vi "UHR-Fleezers Control (host) - 12.1_Jonathan.vi"() -> ()   [LabVIEW 2012] (continued)
          tunnel: [w1121] -> w1086
          tunnel: w1085 -> [w1121]
          tunnel: [w1125] -> w1087
          tunnel: w1086 -> [w1125]
          tunnel: w1087 -> [w1127]
          frame #0 {
            n678 = property on="Trap Delta (MHz)" class="DigNum (strict)"("Val(Sgnl)"="Trap Delta Before Moving") -> ()  [unwired: 2 in, 2 out]
          }
          frame #1 {
            n679 = local read "Saved Stage Positions"() -> (w1098:dbl[][])
            n680 = local write "FB Trap Pos Offset"(0.0 ("FB Trap Pos Offset")) -> ()
            n681 = property on="Trap Pos. FB Offset Factor" class="DigNum (strict)"("Val(Sgnl)"=i64 0 ("Value (Signaling)")) -> ()  [unwired: 2 in, 2 out]
            n682 = local write "Stage Moving"(TRUE ("Stage Moving")) -> ()
            n683 = call "move to saved stage position.vi"("error in"=w1095, "Stage VISA resource name in"=w1096, "Position"="Stage Position To Establish FB", "Saved Stage Positions"=w1098) -> ("error out"=w1094:errorcluster)  [unwired: 1 out]
            n684 = local write "Stage Control Serial Error"(w1094) -> ()
          }
          frame #2 {
            n685 = call <vilib>:"Beep.vi"() -> ()  [unwired: 3 in, 9 out]
            n686 = Multiply(x="Wait (s)", y=u32 1000 ("milliseconds to wait")) -> (x*y=w1104:u32)
            n687 = property on="Trap Delta (MHz)" class="DigNum (strict)"("Val(Sgnl)"="Starting \nTrap Delta (MHz)") -> ()  [unwired: 2 in, 2 out]
            n688 = local write "Stage Moving"(FALSE ("Stage Moving")) -> ()
            n689 = Wait (ms)(milliseconds to wait=w1104) -> ()  [unwired: 1 out]
            n690 = property on="Tab Control 2" class="TabCtl (strict)"("Val(Sgnl)"=T7."Feedback on Trap Position" ("Value (Signaling)")) -> ()  [unwired: 2 in, 2 out]
            n691 = property on="Tab Control" class="TabCtl (strict)"("Val(Sgnl)"=T27."Trap Control (RF)" ("Value (Signaling)")) -> ()  [unwired: 2 in, 2 out]
          }
          frame #3 {
            n692 = property on="Set Reading to\nSetpoint" class="Bool (strict)"("Val(Sgnl)"=TRUE ("Value (Signaling)")) -> ()  [unwired: 2 in, 2 out]
            n693 = Wait (ms)(milliseconds to wait=u32 500) -> ()  [unwired: 1 out]
          }
          frame #4 {
            n694 = property on="Trap Pos. FB ON" class="Bool (strict)"("Val(Sgnl)"=TRUE ("Value (Signaling)")) -> ()  [unwired: 2 in, 2 out]
            n695 = Wait (ms)(milliseconds to wait=u32 250) -> ()  [unwired: 1 out]
          }
          frame #5 {
            n696 = case shown="False" "Trap Trig Fl." {
              frame False {
                n697 = case shown="True" "Green ON after FB ON?" {
                  selector: "Green ON after FB ON?" -> [_ w1120]
                  frame False {
                  }
                  frame True {
                    n698 = property on="Green Laser ON/Interlacing" class="Bool (strict)"("Val(Sgnl)"=w1120) -> ()  [unwired: 2 in, 2 out]
                  }
                }
              }
              frame True {
              }
            }
            n699 = case shown="True" "Remove Action Offset" {
              tunnel: TRUE ("Value (Signaling)") -> [w1117 w1118]
              frame False {
                n700 = property on="Remove Unwinding Offset" class="Bool (strict)"("Val(Sgnl)"=w1117) -> ()  [unwired: 2 in, 2 out]
              }
              frame True {
                n701 = property on="Remove Action Offset" class="Bool (strict)"("Val(Sgnl)"=w1118) -> ()  [unwired: 2 in, 2 out]
              }
            }
            n702 = Wait (ms)(milliseconds to wait=u32 250) -> ()  [unwired: 1 out]
          }
          frame #6 {
            n703 = property on="Start Saving" class="Bool (strict)"("Val(Sgnl)"=TRUE ("Value (Signaling)")) -> ()  [unwired: 2 in, 2 out]
            n704 = Wait (ms)(milliseconds to wait=u32 5000) -> ()  [unwired: 1 out]
          }
          frame #7 {
            w1124 = TRUE ("Value (Signaling)")
            n705 = property on="Rem fb disp offset" class="Bool (strict)"("Val(Sgnl)"=w1124) -> ()  [unwired: 2 in, 2 out]
            n706 = property on="Remove Offset" class="Bool (strict)"("Val(Sgnl)"=w1124) -> ()  [unwired: 2 in, 2 out]
            n707 = Wait (ms)(milliseconds to wait=u32 100) -> ()  [unwired: 1 out]
          }
          frame #8 {
            n708 = case shown="True" w1127 {
              frame False {
              }
              frame True {
                n709 = local write "Trap Trig. Fl."(TRUE ("Value (Signaling)")) -> ()
              }
            }
          }
          frame #9 {
            n710 = case shown="True" "Start dipping after?" {
              frame False {
              }
              frame True {
                n711 = flat-sequence {
                  frame #0 {
                    n712 = Multiply(x="Delay before dipping (s)", y=1000.0) -> (x*y=w1131:dbl)
                    n713 = Wait (ms)(milliseconds to wait=w1131) -> ()  [unwired: 1 out]
                  }
                  frame #1 {
                    n714 = property on="Dip for Protein" class="Bool (strict)"("Val(Sgnl)"=TRUE ("Value (Signaling)")) -> ()  [unwired: 2 in, 2 out]
                    n715 = local write "Scripts"(T2."Dipping" ("Scripts")) -> ()
                  }
                }
              }
            }
          }
        }
      }
      event "Fixed Traps Data\nScript": Value Change {
        n716 = event-data() -> ()  [unwired: 1 in, 5 out]
        n717 = flat-sequence {
          frame #0 {
            n718 = case shown="True" "Green ON" {
              frame False {
              }
              frame True {
                n719 = property on="Green Laser ON/Interlacing" class="Bool (strict)"("Val(Sgnl)"=TRUE) -> ()  [unwired: 2 in, 2 out]
              }
            }
            n720 = local write "Offset (nm)"(0.0 ("Offset (nm)")) -> ()
            n721 = property on="Sample Channel\nFlow" class="Bool (strict)"("Val(Sgnl)"=FALSE ("Value (Signaling)")) -> ()  [unwired: 2 in, 2 out]
            n722 = property on="Trap Delta (MHz)" class="DigNum (strict)"("Val(Sgnl)"="Fixed Traps Trap Delta (MHz)") -> ()  [unwired: 2 in, 2 out]
          }
          frame #1 {
            n723 = Wait (ms)(milliseconds to wait=u32 1000) -> ()  [unwired: 1 out]
          }
          frame #2 {
            n724 = local write "Start Saving"(TRUE ("Start Saving")) -> ()
          }
          frame #3 {
            n725 = local read "Bead Sep. Int. Time (s)"() -> (w1142:dbl)
            n726 = Multiply(x=w1142, y=1000.0) -> (x*y=w1144:dbl)
            n727 = Wait (ms)(milliseconds to wait=w1144) -> ()  [unwired: 1 out]
          }
          frame #4 {
            n728 = property on="Remove Offset" class="Bool (strict)"("Val(Sgnl)"=TRUE ("Value (Signaling)")) -> ()  [unwired: 2 in, 2 out]
          }
          frame #5 {
            n729 = property on="Dip for Protein" class="Bool (strict)"("Val(Sgnl)"="Start dipping after?") -> ()  [unwired: 2 in, 2 out]
          }
        }
      }
      event "Got DNA bead": Value Change {
        n730 = event-data() -> ()  [unwired: 1 in, 5 out]
        n731 = flat-sequence {
          frame #0 {
            n732 = local read "Daq spot flow on"() -> (w1149:bool)
            n733 = case shown="True" w1149 {
              frame False {
              }
              frame True {
                n734 = property on="Sample Channel\nFlow" class="Bool (strict)"("Val(Sgnl)"=TRUE ("Value (Signaling)")) -> ()  [unwired: 2 in, 2 out]
              }
            }
            n735 = property on="Got DNA bead" class="Bool"("Key Focus"=FALSE) -> ()  [unwired: 2 in, 2 out]
          }
          frame #1 {
            n736 = property on="Inject Pump 1" class="Bool (strict)"("Val(Sgnl)"=FALSE ("Value (Signaling)")) -> ()  [unwired: 2 in, 2 out]
          }
          frame #2 {
            n737 = property on="Cal/Data Acq. Spot" class="Bool (strict)"("Val(Sgnl)"=TRUE ("Value (Signaling)")) -> ()  [unwired: 2 in, 2 out]
          }
        }
      }
      event "Take Stepping Data": Value Change {
        n738 = event-data() -> ()  [unwired: 1 in, 5 out]
        n739 = local read "Save ave N"() -> (w1161:dbl)
        n740 = flat-sequence {
          tunnel: w1161 -> [w1163]
          tunnel: [w1163] -> w1156
          tunnel: [w1165] -> w1157
          tunnel: w1156 -> [w1165]
          tunnel: [w1167] -> w1158
          tunnel: w1157 -> [w1167]
          tunnel: [w1170] -> w1159
          tunnel: w1158 -> [w1170]
          tunnel: [w1172] -> w1160
          tunnel: w1159 -> [w1172]
          tunnel: [w1174] -> w1154
          tunnel: w1160 -> [w1174]
          tunnel: w1154 -> [w1177]
          tunnel: [w1177] -> w1153
          tunnel: w1153 -> [w1178]
          tunnel: [w1178] -> w1155
          tunnel: w1155 -> [w1184]
          frame #0 {
            n741 = property on="Save ave N" class="DigNum (strict)"("Val(Sgnl)"="Save ave factor") -> ()  [unwired: 2 in, 2 out]
          }
          frame #1 {
            n742 = Wait (ms)(milliseconds to wait=u32 100) -> ()  [unwired: 1 out]
          }
          frame #2 {
            n743 = local read "Offset 2 Start (MHz)"() -> (w1169:dbl)
            n744 = property on="Saved AOD Raster Scan Parameter Sets" class="Arr (strict)"("Index Values"=u32[] [2]) -> ()  [unwired: 2 in, 2 out]
            n745 = property on="Trap Delta (MHz)" class="DigNum (strict)"("Val(Sgnl)"=w1169) -> ()  [unwired: 2 in, 2 out]
          }
          frame #3 {
            n746 = property on="Load parameters" class="Bool (strict)"("Val(Sgnl)"=TRUE ("Value (Signaling)")) -> ()  [unwired: 2 in, 2 out]
          }
          frame #4 {
            n747 = Wait (ms)(milliseconds to wait=u32 100) -> ()  [unwired: 1 out]
          }
          frame #5 {
            n748 = property on="Trap Raster Scan" class="Bool (strict)"("Val(Sgnl)"=TRUE ("Value (Signaling)")) -> ()  [unwired: 2 in, 2 out]
          }
          frame #6 {
            n749 = Wait (ms)(milliseconds to wait=u32 1000) -> ()  [unwired: 1 out]
          }
          frame #7 {
            n750 = while {
              stop <- w1181 stop-if-true
              n751 = local read "Raster Scanning..."() -> (w1183:bool)
              n752 = local read "Saving..."() -> (w1182:bool)
              n753 = Not(x=w1182) -> (.not. x?=w1179:bool)
              n754 = Not(x=w1183) -> (.not. x?=w1180:bool)
              n755 = And(x=w1180, y=w1179) -> (x .and. y?=w1181:bool)
            }
          }
          frame #8 {
            n756 = property on="Save ave N" class="DigNum (strict)"("Val(Sgnl)"=w1184) -> ()  [unwired: 2 in, 2 out]
          }
        }
      }
      event "Step Size (nm)": Value Change {
        n757 = event-data() -> ()  [unwired: 1 in, 5 out]
        n758 = flat-sequence {
          frame #0 {
            n759 = property on="Saved AOD Raster Scan Parameter Sets" class="Arr (strict)"("Index Values"=u32[] [1]) -> ()  [unwired: 2 in, 2 out]
          }
          frame #1 {
            n760 = Multiply(x="N Steps", y="Step Size (nm)") -> (x*y=w1186:dbl)
            n761 = property on="Scan Speed AOD (nm/s) 2" class="DigNum (strict)"("Value"="Step Size (nm)") -> ()  [unwired: 2 in, 2 out]
            n762 = property on="Step Size AOD (nm) 2" class="DigNum (strict)"("Value"="Step Size (nm)") -> ()  [unwired: 2 in, 2 out]
            n763 = property on="Scan Range AOD (nm) 2" class="DigNum (strict)"("Value"=w1186) -> ()  [unwired: 2 in, 2 out]
          }
        }
      }
      event "Take Detection Laser\nImage": Value Change {
        n764 = event-data() -> ()  [unwired: 1 in, 5 out]
        n765 = flat-sequence {
          tunnel: [w1214] -> w1204
          tunnel: [w1213] -> w1197
          tunnel: [w1212] -> w1189
          tunnel: [w1217] -> w1205
          tunnel: w1204 -> [w1217]
          tunnel: [w1216] -> w1198
          tunnel: w1197 -> [w1216]
          tunnel: [w1215] -> w1190
          tunnel: w1189 -> [w1215]
          tunnel: [w1221] -> w1206
          tunnel: w1205 -> [w1221]
          tunnel: [w1220] -> w1199
          tunnel: w1198 -> [w1220]
          tunnel: [w1219] -> w1191
          tunnel: w1190 -> [w1219]
          tunnel: [w1227] -> w1207
          tunnel: w1206 -> [w1227]
          tunnel: [w1226] -> w1200
          tunnel: w1199 -> [w1226]
          tunnel: [w1225] -> w1192
          tunnel: w1191 -> [w1225]
          tunnel: [w1231] -> w1208
          tunnel: w1207 -> [w1231]
          tunnel: [w1230] -> w1201
          tunnel: w1200 -> [w1230]
          tunnel: [w1229] -> w1193
          tunnel: w1192 -> [w1229]
          tunnel: [w1235] -> w1209
          tunnel: w1208 -> [w1235]
          tunnel: [w1234] -> w1202
          tunnel: w1201 -> [w1234]
          tunnel: [w1233] -> w1194
          tunnel: w1193 -> [w1233]
          tunnel: [w1239] -> w1210
          tunnel: w1209 -> [w1239]
          tunnel: [w1238] -> w1203
          tunnel: w1202 -> [w1238]
          tunnel: [w1237] -> w1195
          tunnel: w1194 -> [w1237]
          tunnel: w1210 -> [w1245]
          tunnel: w1203 -> [w1244]
          tunnel: [w1242] -> w1196
          tunnel: w1195 -> [w1242]
          tunnel: w1196 -> [w1246]
          frame #0 {
            n766 = local read "Green Laser ON/Interlacing"() -> (w1214:bool)
            n767 = local read "Green laser mode"() -> (w1213:enum32{"Laser ON", "Laser OFF", "Interlace"})
            n768 = local read "Green FB On/Off"() -> (w1212:bool)
          }
          frame #1 {
            n769 = property on="Green FB On/Off" class="Bool (strict)"("Val(Sgnl)"=FALSE ("Value (Signaling)")) -> ()  [unwired: 2 in, 2 out]
          }
          frame #2 {
            n770 = property on="Green Laser ON/Interlacing" class="Bool (strict)"("Val(Sgnl)"=TRUE ("Value (Signaling)")) -> ()  [unwired: 2 in, 2 out]
            n771 = property on="Flip Green Filter" class="Bool (strict)"("Val(Sgnl)"=TRUE ("Value (Signaling)")) -> ()  [unwired: 2 in, 2 out]
            n772 = property on="Green laser mode" class="RadioBtnsControl (strict)"("Val(Sgnl)"=enum32{"Laser ON", "Laser OFF", "Interlace"}."Laser ON" ("Value (Signaling)")) -> ()  [unwired: 2 in, 2 out]
          }
          frame #3 {
            n773 = Wait (ms)(milliseconds to wait=u32 500) -> ()  [unwired: 1 out]
          }
          frame #4 {
            n774 = property on="Confocal Image" class="Bool (strict)"("Val(Sgnl)"=TRUE ("Value (Signaling)")) -> ()  [unwired: 2 in, 2 out]
          }
          frame #5 {
            n775 = Wait (ms)(milliseconds to wait=u32 2000) -> ()  [unwired: 1 out]
          }
          frame #6 {
            n776 = while {
              stop <- w1240 stop-if-true
              n777 = local read "Saving..."() -> (w1241:bool)
              n778 = Not(x=w1241) -> (.not. x?=w1240:bool)
            }
          }
          frame #7 {
            n779 = property on="Flip Green Filter" class="Bool (strict)"("Val(Sgnl)"=TRUE ("Value (Signaling)")) -> ()  [unwired: 2 in, 2 out]
            n780 = property on="Green Laser ON/Interlacing" class="Bool (strict)"("Val(Sgnl)"=w1245) -> ()  [unwired: 2 in, 2 out]
            n781 = property on="Green laser mode" class="RadioBtnsControl (strict)"("Val(Sgnl)"=w1244) -> ()  [unwired: 2 in, 2 out]
          }
          frame #8 {
            n782 = property on="Green FB On/Off" class="Bool (strict)"("Val(Sgnl)"=w1246) -> ()  [unwired: 2 in, 2 out]
          }
        }
      }
      event "Stop All": Value Change {
        n783 = event-data() -> ()  [unwired: 1 in, 5 out]
        n784 = local read "Stop All"() -> (w1247:bool)
      }
    }
    n785 = node-c288() -> ()  [unwired: 1 in, 1 out]
  }
  n786 = node-c288(3 ("Processor")) -> (w97:T22)  [unwired: 3 out]
  n787 = flat-sequence "Video" {
    tunnel: [w1257] -> w87
    tunnel: w87 -> [w1297]
    frame #0 {
      n788 = while {
        stop <- w1249 continue-if-true
        n789 = call "Close Video Capture.vi"() -> ("error code OUT"=w1251:i32)
        n790 = Equal?(x=w1251, y=0) -> (x = y?=w1249:bool)
      }
      n791 = local write "Stop All"(FALSE ("Stop All")) -> ()
    }
    frame #1 {
      n792 = call "DMR_Init.vi"() -> ()  [unwired: 3 out]
    }
    frame #2 {
      w1252 = "DE245428202"  # MSU fleezers card #
      (unwired) "DE019116701"  # Illinois fleezers card #
      # "Setting the destination format to Mono8 makes sure that the image can be displayed in the intensity plot."
      n793 = call "DMR_GetDevice.vi"("search string IN"=w1252) -> ("device handle OUT"=w1275:i32)  [unwired: 4 in, 2 out]
      n794 = call "DMR_OpenDevice.vi"("device handle IN"=w1275) -> ("driver handle OUT"=w1258:i32)  [unwired: 4 out]
      n795 = call "DMR_FindList.vi"("flags IN"=u32 0 ("flags"), "list name IN"="" ("String"), "list type IN"=T28."camera descriptions", "driver handle IN"=w1258) -> ("list handle OUT"=w1261:i32)  [unwired: 2 out]
      n796 = call "DMR_FindList.vi"("flags IN"=u32 0 ("flags"), "list name IN"="Base", "list type IN"=T28."setting", "driver handle IN"=w1258) -> ("list handle OUT"=w1259:i32)  [unwired: 2 out]
      n797 = call "OBJ_GetHandle.vi"("object name IN"="VideoStandard", "list handle IN"=w1261) -> ("object handle OUT"=w1255:i32)  [unwired: 3 out]
      n798 = call "OBJ_GetHandle.vi"("object name IN"="PixelFormat", "list handle IN"=w1259) -> ("object handle OUT"=w1269:i32)  [unwired: 3 out]
      n799 = call "OBJ_SetS.vi"("value index IN"=0, "value IN"="NTSC M", "object handle IN"=w1255) -> ()  [unwired: 2 out]
      n800 = call "OBJ_SetS.vi"("value index IN"=0, "value IN"="Mono8" ("value"), "object handle IN"=w1269) -> ()  [unwired: 2 out]
      n801 = call "OBJ_GetHandle.vi"("object name IN"="VideoChannel", "list handle IN"=w1259) -> ("object handle OUT"=w1265:i32)  [unwired: 3 out]
      n802 = while {
        tunnel: [w1279] -> w1257
        tunnel: w1258 -> [w1276]
        stop <- w1277 continue-if-true
        n803 = call "DMR_ImageRequestSingle.vi"("request control IN"=0, "driver handle IN"=w1276) -> ("error code OUT"=w1278:i32, "driver handle OUT"=w1279:i32)  [unwired: 2 out]
        n804 = Equal To 0?(x=w1278) -> (x = 0?=w1277:bool)
      }
      n805 = call "OBJ_SetI.vi"("value index IN"=0, "value IN"=3 ("Video channel"), "object handle IN"=w1265) -> ()  [unwired: 2 out]
    }
    frame #3 {
      w1285 = T18 0 items=["Grayscale (U8)", "Grayscale (I16)", "Grayscale (SGL)", "Complex (CSG)", "RGB (U32)", "HSL (U32)", "RGB (U64)"] ("Image Type")
      w1293 = T18 0 items=["Grayscale (U8)", "Grayscale (I16)", "Grayscale (SGL)", "Complex (CSG)", "RGB (U32)", "HSL (U32)", "RGB (U64)"] ("Image Type")
      n806 = for "Create Greyscale map" {
        N: 256 -> [_]
        tunnel: [w1299] -> w1282 mode=indexing
        workers-P: _ -> [_]
        i -> [w1302]
        n807 = To Unsigned Byte Integer(number=w1302) -> (unsigned 8bit integer=w1298:u8)
        n808 = Join Numbers(hi=w1298, lo=w1298) -> ((hi.lo)=w1301:u16)
        n809 = Join Numbers(hi=w1298, lo=w1298) -> ((hi.lo)=w1300:u16)
        n810 = Join Numbers(hi=w1301, lo=w1300) -> ((hi.lo)=w1299:u32)
      }
      n811 = call "IMAQ Create"("Image Name"="Scaled video", "Image Type"=w1285) -> ("New Image"=w1284:T3)  [unwired: 2 in, 2 out]
      n812 = call "IMAQ Create"("Image Name"="Main video", "Image Type"=w1293) -> ("New Image"=w1294:T3)  [unwired: 2 in, 2 out]
      n813 = node-c288(0 ("Processor")) -> (w1292:T22)  [unwired: 3 out]
      n814 = Initialize Array(u32 0 ("Window Number (0...15)"), 480 ("dimension size"), 640 ("dimension size")) -> (w1287:u32[][])
      n815 = timed-loop {
        tunnel: w1297 -> [w1319]
        tunnel: [w1318] -> w1296
        tunnel: w1294 -> [w1317]
        timing: w1292 -> [_]
        timing-out: [_] -> w1291
        tunnel: w1287 -> [w1306]
        tunnel: w1284 -> [w1304]
        tunnel: w1282 -> [w1303]
        stop <- w1305 stop-if-true
        # "This block performs the \nactual image capture."
        n816 = node-c288() -> ()  [unwired: 2 out]
        n817 = local read "Stop All"() -> (w1305:bool)
        n818 = Reciprocal(x="Video Capture Rate (Hz)") -> (1/x=w1309:dbl)
        n819 = Multiply(x=w1309, y=1000.0) -> (x*y=w1307:dbl)
        n820 = call "DMR_ImageRequestWaitFor.vi"("queue number IN"=0, "timeout(ms) IN"=500, "driver handle IN"=w1319) -> ("error code OUT"=w1323:i32, "request number OUT"=w1320:i32, "driver handle OUT"=w1321:i32)
        n821 = feedback #1(T29 refnum ("Avi Refnum")) -> (w1311:T29)
        n822 = case shown="True" "New Video File" {
          tunnel: [T29 refnum ("Avi Refnum") w1340] -> w1313
          tunnel: [FALSE TRUE] -> w1314
          tunnel: w1311 -> [_ w1336]
          frame False {
          }
          frame True {
            n823 = call "Create new save file.vi"("Ext"=".avi" ("string"), "Index In"="Video Index") -> ("Path Out"=w1332:path, "Index Out"=w1333:dbl)  [unwired: 1 in]
            "Path Out" <- w1332
            n824 = Not Equal?(x=w1336, y=T29 refnum ("Avi Refnum")) -> (x != y?=w1337:bool)
            n825 = Increment(x=w1333) -> (x+1=w1342:dbl)
            n826 = case shown="True" w1337 {
              tunnel: w1336 -> [_ w1343]
              frame False {
              }
              frame True {
                n827 = call "IMAQ AVI Close"("Avi Refnum"=w1343) -> ()  [unwired: 1 in, 10 out]
              }
            }
            n828 = local write "Video Index"(w1342) -> ()
            n829 = call "IMAQ AVI Create"("Frames Per Second"=u32 30, "AVI Path"=w1332) -> ("Avi Refnum"=w1340:T29)  [unwired: 5 in, 4 out]
          }
        }
        n830 = Equal To 0?(x=w1323) -> (x = 0?=w1322:bool)
        n831 = Select(t=w1313, s=w1314, f=w1311) -> (s? t:f=w1312:T29)
        n832 = feedback-in #1(w1312) -> ()
        n833 = case shown="True" w1322 {
          tunnel: w1321 -> [w1344 w1369]
          tunnel: w1320 -> [_ w1368]
          tunnel: [w1344 w1365] -> w1318
          tunnel: w1317 -> [_ w1349]
          tunnel: w1306 -> [_ w1353]
          tunnel: w1312 -> [_ w1351]
          tunnel: w1304 -> [_ w1346]
          tunnel: w1303 -> [_ w1345]
          frame False {
          }
          frame True {
            w1359 = u32 0 ("X-offset IN")
            n834 = call "DMR_GetImageRequestBufferData.vi"("driver handle IN"=w1369, "request number IN"=w1368) -> ("width OUT"=w1358:i32, "height OUT"=w1357:i32, "driver handle OUT"=w1364:i32, "request number OUT"=w1363:i32, "bytes per pixel OUT"=w1360:i32)  [unwired: 13 out]
            n835 = call "DMR_GetImageRequestBufferImageData.vi"("driver handle IN"=w1364, "request number IN"=w1363, "bytes per pixel IN"=w1360, "X-offset IN"=w1359, "Y-offset IN"=w1359, "height IN"=w1357, "width IN"=w1358) -> ("driver handle OUT"=w1362:u32, "request number OUT"=w1361:u32, "image OUT"=w1354:u32[][])  [unwired: 10 out]
            n836 = call "DMR_ImageRequestUnlock.vi"("request number IN"=w1361, "driver handle IN"=w1362) -> ("driver handle OUT"=w1367:i32)  [unwired: 1 in, 2 out]
            n837 = case shown="True" "Averaging" {
              tunnel: w1354 -> [w1405 w1410]
              tunnel: [w1405 w1409] -> w1350
              tunnel: w1353 -> [_ w1407]
              frame False {
              }
              frame True {
                (unwired) 1
                w1415 = 1
                n838 = feedback #2(w1407) -> (w1406:u32[][])
                n839 = Add(x=w1410, y=w1406) -> (x+y=w1411:u32[][])
                n840 = Select(t=w1407, s="Reset Averaging", f=w1411) -> (s? t:f=w1413:u32[][])
                n841 = feedback-in #2(w1413) -> ()
                n842 = feedback #3(w1415) -> (w1408:i32)
                n843 = Divide(x=w1411, y=w1408) -> (x/y=w1412:dbl[][])
                n844 = Increment(x=w1408) -> (x+1=w1416:i32)
                n845 = To Unsigned Long Integer(number=w1412) -> (unsigned 32bit integer=w1409:u32[][])
                n846 = Select(t=w1415, s="Reset Averaging", f=w1416) -> (s? t:f=w1414:i32)
                n847 = feedback-in #3(w1414) -> ()
              }
            }
            n848 = call "DMR_ImageRequestSingle.vi"("request control IN"=0, "driver handle IN"=w1367) -> ("driver handle OUT"=w1365:i32)  [unwired: 3 out]
            n849 = disable-structure shown="Disabled" {
              disable-tunnel: w1350 -> [w1382 _]
              disable-tunnel: w1346 -> [w1381 _]
              frame Disabled {
                n850 = To Double Precision Float(number=w1382) -> (double precision float=w1380:dbl[][])
                n851 = In Range and Coerce(upper limit="Intensity Upper", x=w1380, lower limit="Intensity Lower") -> (coerced(x)=w1379:dbl[][])  [unwired: 1 out]
                n852 = Subtract(x="Intensity Upper", y="Intensity Lower") -> (x-y=w1376:dbl)
                n853 = Subtract(x=w1379, y="Intensity Lower") -> (x-y=w1377:dbl[][])
                n854 = Divide(x=w1377, y=w1376) -> (x/y=w1378:dbl[][])
                n855 = Multiply(x=255.0, y=w1378) -> (x*y=w1374:dbl[][])
                n856 = To Unsigned Byte Integer(number=w1374) -> (unsigned 8bit integer=w1383:u8[][])
                n857 = call "IMAQ ArrayToImage"("Image Pixels (U8)"=w1383, "Image"=w1381) -> ("Image Out"=w1370:T3)  [unwired: 4 in, 5 out]
                n858 = First Call?() -> (First Call?: T/F=w1371:bool)
                n859 = case shown="True" w1371 {
                  tunnel: w1370 -> [w1384 w1395]
                  frame False {
                    n860 = flat-sequence {
                      tunnel: w1384 -> [w1390]
                      frame #0 {
                        w1387 = FALSE ("Get/Set Status? (Set)")
                        w1386 = 0 ("Window Number (0...15)")
                        n861 = call "IMAQ WindSize"("Get/Set Status? (Set)"=w1387, "Window Number"=w1386) -> ("Width & Height out"=→"Window Size":cluster{"Width":i32, "Height":i32})  [unwired: 4 in, 2 out]
                        n862 = call "IMAQ WindMove"("Window Number (0...15)"=w1386, "Get/Set Status? (Set)"=w1387) -> ("Coordinates (screen)"=→"Window Position":cluster{"X Position":i32, "Y Position":i32})  [unwired: 3 in, 1 out]
                        n863 = call "IMAQ WindDraw"("Resize to Image Size? (Y)"=FALSE, "Window Number (0...15)"=w1386, "Image"=w1390) -> ()  [unwired: 7 in, 2 out]
                      }
                      frame #1 {
                        n864 = call "IMAQ WindZoom 2"("Center Point"="Center Point", "Zoom to Fit? (False)"=FALSE, "Zoom Factor"="Zoom Factor") -> ()  [unwired: 5 in, 4 out]
                      }
                    }
                  }
                  frame True {
                    n865 = flat-sequence {
                      tunnel: w1395 -> [w1398]
                      tunnel: [w1396] -> w1394
                      tunnel: w1394 -> [w1400]
                      frame #0 {
                        w1397 = TRUE ("Resize to Image Size? (Y)")
                        w1396 = 0 ("Window Number (0...15)")
                        n866 = call "IMAQ WindNonTearing"("Window Number"=w1396, "NonTearing? (True)"=w1397) -> ()  [unwired: 8 in, 2 out]
                        n867 = call "IMAQ WindDraw"("Resize to Image Size? (Y)"=w1397, "Window Number (0...15)"=w1396, "Image"=w1398) -> ()  [unwired: 7 in, 2 out]
                      }
                      frame #1 {
                        n868 = call "IMAQ WindSize"("Scrollbars? (N)"=FALSE, "Width & Height"="Initial Window Size", "Window Number"=w1400) -> ()  [unwired: 3 in, 3 out]
                        n869 = call "IMAQ WindMove"("Window Number (0...15)"=w1400, "Coordinates (screen)"="Initial Window Position") -> ()  [unwired: 3 in, 2 out]
                      }
                    }
                  }
                }
              }
              frame Enabled {
              }
            }
            n870 = To Unsigned Byte Integer(number=w1350) -> (unsigned 8bit integer=w1348:u8[][])
            n871 = call "IMAQ ArrayToImage"("Image Pixels (U8)"=w1348, "Image"=w1349) -> ("Image Out"=w1347:T3)  [unwired: 4 in, 5 out]
            "Primary Video Display" <- w1347
            n872 = case shown="True" "Save Video" {
              tunnel: w1351 -> [_ w1404]
              tunnel: w1347 -> [_ w1403]
              frame False {
              }
              frame True {
                n873 = call "IMAQ AVI Write Frame"("Image"=w1403, "Avi Refnum"=w1404) -> ()  [unwired: 2 in, 8 out]
              }
            }
            n874 = case shown="True" "Save Image" {
              tunnel: w1348 -> [_ w1419]
              tunnel: w1345 -> [_ w1418]
              frame False {
              }
              frame True {
                n875 = call <vilib>:"Flatten Pixmap.vi"("colors"=w1418, "8-bit pixmap"=w1419) -> ("image data"=w1425:T30)  [unwired: 4 in, 5 out]
                n876 = call "Create new save file.vi"("Insert"="video_frame_" ("string"), "Ext"=".bmp" ("string"), "Index In"="Image Index") -> ("Path Out"=w1421:path, "Index Out"=w1426:dbl)
                n877 = Increment(x=w1426) -> (x+1=w1420:dbl)
                n878 = local write "Image Index"(w1420) -> ()
                n879 = call <vilib>:"Write BMP File.vi"("image data"=w1425, "path to BMP file"=w1421) -> ()  [unwired: 1 in, 9 out]
              }
            }
          }
        }
        n880 = node-c288(w1307) -> ()  [unwired: 1 out]
      }
      n881 = node-c288(w1291) -> ()  [unwired: 1 out]
      n882 = call "DMR_CloseDevice.vi"("driver handle IN"=w1296) -> ()  [unwired: 1 in, 4 out]
    }
    frame #4 {
      n883 = call "DMR_Close.vi"() -> ()  [unwired: 1 out]
    }
  }
  n884 = timed-loop "Acquire Data" {
    tunnel: w8 -> [w1727]
    tunnel: w57 -> [w1726]
    tunnel: [w1756] -> w276
    tunnel: [w1751] -> w274
    timing: w181 -> [_]
    timing-out: [_] -> w180
    tunnel: w76 -> [w1564]
    stop <- "Stop All" stop-if-true
    w1479 = "Initialize"
    w1549 = "NI_ChannelName" ("name")
    n885 = node-c288() -> ()  [unwired: 2 out]
    n886 = First Call?() -> (First Call?: T/F=w1514:bool)
    n887 = Or(x="Reset", y=w1514) -> (x .or. y?=w1515:bool)
    n888 = local read "Flushing P1"() -> (w1434:bool)
    n889 = case "Reset data stream" shown="True" w1515 {
      tunnel: w1727 -> [w2731 w2739]
      tunnel: w1726 -> [w2730 w2738]
      tunnel: [w2731 w2733] -> w1722
      tunnel: [w2730 w2732] -> w1721
      frame False {
      }
      frame True {
        w2736 = TRUE ("AI to FIFO")
        n890 = local write "Overflow (data lost)"(FALSE ("Overflow (data lost)")) -> ()
        n891 = call "reset FPGA DMA.vi"("error in"=w2738, "FPGA VI Reference In"=w2739) -> ("error out"=w2734:errorcluster, "FPGA VI Reference Out"=w2735:T20)
        n892 = xnode "Read/Write Control"("FPGA VI Reference In"=w2735, "error in"=w2734, "AI to FIFO"=w2736, "APD to FIFO"=w2736) -> ("FPGA VI Reference Out"=w2733:T20, "error out"=w2732:errorcluster)
      }
    }
    n893 = case shown="True" w1434 {
      frame False {
      }
      frame True {
        n894 = local read "Flush rate (uL/m) P1"() -> (w1772:dbl)
        n895 = local read "HP1 Flush Time (s)"() -> (w1781:dbl)
        n896 = local read "DMA Update Period (s)"() -> (w1775:dbl)
        n897 = Divide(x=w1772, y=60.0) -> (x/y=w1773:dbl)
        n898 = Divide(x=w1781, y=w1775) -> (x/y=w1770:dbl)
        n899 = feedback #4(0) -> (w1779:i32)
        n900 = Increment(x=w1779) -> (x+1=w1769:i32)
        n901 = Greater?(x=w1769, y=w1770) -> (0:w1778:bool)
        n902 = Compound Arithmetic op=MULTIPLY(w1775, w1769, w1773) -> (→"P1 Flush Volume (uL)":dbl)
        n903 = Divide(x=w1769, y=w1770) -> (x/y=→"P1 Flushing Bar":dbl)
        n904 = case shown="True" w1778 {
          tunnel: w1769 -> [w1782 _]
          tunnel: [w1782 0] -> w1777
          frame False {
          }
          frame True {
            w1783 = FALSE ("Flushing P1")
            n905 = local write "Inject Pump 1"(w1783) -> ()
            n906 = local write "Flushing P1"(w1783) -> ()
            n907 = property on="Clear Volume P1" class="Bool (strict)"("Val(Sgnl)"=TRUE ("Value (Signaling)")) -> ()  [unwired: 2 in, 2 out]
          }
        }
        n908 = feedback-in #4(w1777) -> ()
      }
    }
    n909 = Or(x="Start AOD Scan", y="Trap Raster Scan") -> (x .or. y?=w1672:bool)
    n910 = case "Start AOM raster scan" shown="True" w1672 {
      tunnel: w1722 -> [w2581 w2591]
      tunnel: w1721 -> [w2580 w2590]
      tunnel: [w2581 w2584] -> w1720
      tunnel: [w2580 w2583] -> w1719
      frame False {
      }
      frame True {
        n911 = case shown="True" "Restart DMA? (AOD)" {
          tunnel: [w2629 w2631] -> w2585
          tunnel: [w2628 w2630] -> w2586
          tunnel: w2591 -> [w2629 w2633]
          tunnel: w2590 -> [w2628 w2632]
          frame False {
          }
          frame True {
            n912 = local write "Overflow (data lost)"(FALSE ("Overflow (data lost)")) -> ()
            n913 = call "reset FPGA DMA.vi"("error in"=w2632, "FPGA VI Reference In"=w2633) -> ("error out"=w2630:errorcluster, "FPGA VI Reference Out"=w2631:T20)
          }
        }
        n914 = local write "Trap Raster Scan"(FALSE ("Trap Raster Scan")) -> ()
        n915 = case shown="True" "Move MCL Also?" {
          tunnel: w2586 -> [w2594 w2623]
          tunnel: w2585 -> [w2595 w2624]
          tunnel: [w2593 w2627] -> w2584
          tunnel: [w2592 w2626] -> w2583
          frame False {
            w2596 = TRUE ("AI to FIFO")
            n916 = xnode "Read/Write Control"("FPGA VI Reference In"=w2595, "error in"=w2594, "AI to FIFO"=w2596, "APD to FIFO"=w2596, "Start scan"=w2596) -> ("FPGA VI Reference Out"=w2593:T20, "error out"=w2592:errorcluster)
          }
          frame True {
            w2620 = FALSE ("1D or 2D Scan?")
            w2625 = TRUE ("AI to FIFO")
            # "Count for MCL loop"
            # "N total cycles"
            # "N steps"
            # "V_int"
            n917 = local read "Scan Range (nm)"() -> (w2602:dbl)
            n918 = local read "Number of F/B Scans (AOD)"() -> (w2619:u16)
            n919 = Sign(1:w2602) -> (0:w2601:dbl)
            n920 = Compound Arithmetic op=MULTIPLY(w2602, "MCL Step Position Ratio", "MCL/AOM Scale Tweak") -> (w2606:dbl)
            n921 = Negate(x=w2601) -> (-x=w2598:dbl)
            n922 = Multiply(x=w2598, y="MCL Step Increment (V_int)") -> (x*y=w2600:dbl)
            n923 = Divide(x=w2606, y="MCL X Cal (nm/V)") -> (x/y=w2612:dbl)
            n924 = Multiply(x=32767.0 ("y"), y=w2612) -> (x*y=w2618:dbl)
            n925 = local read "Total Counts (ticks)"() -> (w2603:u32)
            n926 = local read "Cycles/step (AOD)"() -> (w2614:u64)
            n927 = local read "Scan steps (AOD)"() -> (w2615:u64)
            n928 = Divide(x=w2618, y=10.0) -> (x/y=w2611:dbl)
            n929 = Divide(x=w2611, y="MCL Step Increment (V_int)") -> (x/y=w2609:dbl)
            n930 = Absolute Value(x=w2609) -> (abs(x)=w2597:dbl)
            n931 = Compound Arithmetic op=MULTIPLY(w2615, w2614, w2603) -> (w2610:u64)
            n932 = local write "wait to reset values"(w2625) -> ()
            n933 = local write "MCL Scanning"(w2625) -> ()
            n934 = Divide(x=w2610, y=w2597) -> (x/y=w2607:dbl)
            "MCL Count" <- w2607
            n935 = xnode "Read/Write Control"("FPGA VI Reference In"=w2624, "error in"=w2623, "Scan steps (MCL)"=w2597, "Number of scans (MCL)"=w2619, "Cycles per step (MCL)"=u64 1, "Scan freq.  increment (MCL)"=w2600, "1D or 2D Scan?"=w2620, "MCL Scan Axis"=w2620, "Cont. Scan (MCL)"=w2620, "MCL count"=w2607) -> ("FPGA VI Reference Out"=w2622:T20, "error out"=w2621:errorcluster)
            n936 = xnode "Read/Write Control"("FPGA VI Reference In"=w2622, "error in"=w2621, "AI to FIFO"=w2625, "APD to FIFO"=w2625, "Start scan"=w2625, "Start scan (MCL)"=w2625) -> ("FPGA VI Reference Out"=w2627:T20, "error out"=w2626:errorcluster)
          }
        }
        "Raster Scanning..." <- TRUE ("Scanning...")
      }
    }
    n937 = local read "Flushing P3"() -> (w1435:bool)
    n938 = case "Keep track of when Harvard Pump 3 is done flushing" shown="True" w1435 {
      frame False {
      }
      frame True {
        n939 = local read "Flush rate (uL/m) P3"() -> (w1789:dbl)
        n940 = local read "DMA Update Period (s)"() -> (w1791:dbl)
        n941 = local read "HP3 Flush Time (s)"() -> (w1798:dbl)
        n942 = Divide(x=w1789, y=60.0) -> (x/y=w1787:dbl)
        n943 = feedback #5(0) -> (w1796:i32)
        n944 = Increment(x=w1796) -> (x+1=w1790:i32)
        n945 = Divide(x=w1798, y=w1791) -> (x/y=w1792:dbl)
        n946 = Greater?(x=w1790, y=w1792) -> (0:w1795:bool)
        n947 = Compound Arithmetic op=MULTIPLY(w1791, w1790, w1787) -> (→"P3 Flush Volume (uL)":dbl)
        n948 = case shown="True" w1795 {
          tunnel: w1790 -> [w1799 _]
          tunnel: [w1799 0] -> w1794
          frame False {
          }
          frame True {
            w1800 = FALSE ("Flushing P3")
            n949 = local write "Inject Pump 3"(w1800) -> ()
            n950 = local write "Flushing P3"(w1800) -> ()
            n951 = property on="Clear Volume P3" class="Bool (strict)"("Val(Sgnl)"=TRUE ("Value (Signaling)")) -> ()  [unwired: 2 in, 2 out]
          }
        }
        n952 = feedback-in #5(w1794) -> ()
        n953 = Divide(x=w1790, y=w1792) -> (x/y=→"P3 Flushing Bar":dbl)
      }
    }
    n954 = And(x="Save scans", y=w1672) -> (x .and. y?=w1718:bool)
    n955 = Compound Arithmetic op=OR("Start MCL Scan", "Confocal Image", "Confocal Linescan") -> (w1670:bool)
    n956 = And(x="Save Data (MCL)", y=w1670) -> (x .and. y?=w1717:bool)
    n957 = case "Start MCL raster scan" shown="True" w1670 {
      tunnel: w1720 -> [w2198 w2214]
      tunnel: w1719 -> [w2197 w2213]
      tunnel: [w2198 w2209] -> w1562
      tunnel: [w2197 w2208] -> w1561
      tunnel: [FALSE w2207] -> w1703
      tunnel: "Start MCL Scan" -> [_ w2202]
      tunnel: "Confocal Image" -> [_ w2201]
      tunnel: "Confocal Linescan" -> [_ _]
      frame False {
      }
      frame True {
        w2207 = TRUE
        n958 = case shown="True" "Restart DMA? (MCL)" {
          tunnel: [w2259 w2261] -> w2212
          tunnel: [w2258 w2260] -> w2211
          tunnel: w2214 -> [w2259 w2264]
          tunnel: w2213 -> [w2258 w2263]
          frame False {
          }
          frame True {
            n959 = call "reset FPGA DMA.vi"("error in"=w2263, "FPGA VI Reference In"=w2264) -> ("error out"=w2260:errorcluster, "FPGA VI Reference Out"=w2261:T20)
            n960 = local write "Overflow (data lost)"(FALSE ("Overflow (data lost)")) -> ()
          }
        }
        n961 = case shown="False" w2202 {
          selector: w2202 -> [_ w2218]
          tunnel: w2201 -> [w2217 _]
          tunnel: [w2217 w2218] -> w2200
          frame False {
            n962 = property on="2D or 1D Scan" class="Bool (strict)"("Val(Sgnl)"=w2217) -> ()  [unwired: 2 in, 2 out]
            n963 = property on="Confocal Image" class="Bool (strict)"("Value"=FALSE ("Start Confocal Map")) -> ()  [unwired: 2 in, 2 out]
          }
          frame True {
          }
        }
        n964 = local write "MCL Scanning"(w2207) -> ()
        n965 = local read "AO1"() -> (w2204:dbl)
        n966 = local read "AO2"() -> (w2203:dbl)
        n967 = case shown="True" "Center Scan" {
          tunnel: w2212 -> [w2225 w2257]
          tunnel: w2211 -> [w2224 w2256]
          tunnel: [w2223 w2255] -> w2209
          tunnel: [w2222 w2254] -> w2208
          tunnel: [w2220 w2241] -> w2206
          tunnel: [w2219 w2240] -> w2205
          tunnel: w2204 -> [w2220 w2246]
          tunnel: w2203 -> [w2219 w2249]
          tunnel: w2200 -> [_ _]
          frame False {
            w2221 = TRUE ("AI to FIFO")
            n968 = xnode "Read/Write Control"("FPGA VI Reference In"=w2225, "error in"=w2224, "AI to FIFO"=w2221, "APD to FIFO"=w2221, "Start scan (MCL)"=w2221) -> ("FPGA VI Reference Out"=w2223:T20, "error out"=w2222:errorcluster)
          }
          frame True {
            w2253 = TRUE ("AI to FIFO")
            n969 = local read "Scan steps (MCL)"() -> (w2232:u64)
            n970 = local read "Scan lines (y)"() -> (w2228:u64)
            n971 = local read "Fast Scan Dir"() -> (w2239:bool)
            n972 = local read "Actual MCL Inc (V)"() -> (w2229:dbl)
            n973 = Decrement(x=w2228) -> (x-1=w2227:u64)
            n974 = Decrement(x=w2232) -> (x-1=w2231:u64)
            n975 = Multiply(x=w2229, y=w2227) -> (x*y=w2226:dbl)
            n976 = Divide(x=w2226, y=2.0) -> (x/y=w2236:dbl)
            n977 = Multiply(x=w2229, y=w2231) -> (x*y=w2230:dbl)
            n978 = Divide(x=w2230, y=2.0) -> (x/y=w2235:dbl)
            n979 = Select(t=w2235, s=w2239, f=w2236) -> (s? t:f=w2234:dbl)
            n980 = Select(t=w2236, s=w2239, f=w2235) -> (s? t:f=w2238:dbl)
            n981 = Subtract(x=w2246, y=w2238) -> (x-y=w2237:dbl)
            n982 = Subtract(x=w2249, y=w2234) -> (x-y=w2233:dbl)
            n983 = local read "2D or 1D Scan"() -> (w2251:bool)
            n984 = Not(x=w2239) -> (.not. x?=w2245:bool)
            n985 = Not(x=w2251) -> (.not. x?=w2247:bool)
            n986 = And(x=w2239, y=w2247) -> (x .and. y?=w2248:bool)
            n987 = And(x=w2247, y=w2245) -> (x .and. y?=w2250:bool)
            n988 = Select(t=w2249, s=w2250, f=w2233) -> (s? t:f=w2240:dbl)
            n989 = Select(t=w2246, s=w2248, f=w2237) -> (s? t:f=w2241:dbl)
            n990 = call "Volt to I16.vi"("Voltage In"=w2241) -> ("I16 Voltage Out"=w2244:i16)
            n991 = call "Volt to I16.vi"("Voltage In"=w2240) -> ("I16 Voltage Out"=w2243:i16)
            n992 = xnode "Read/Write Control"("FPGA VI Reference In"=w2257, "error in"=w2256, "AI to FIFO"=w2253, "APD to FIFO"=w2253, "Start scan (MCL)"=w2253, "AO1"=w2244, "AO2"=w2243) -> ("FPGA VI Reference Out"=w2255:T20, "error out"=w2254:errorcluster)
          }
        }
        "Initial Y" <- w2206
        "Initial X" <- w2205
        n993 = local write "Tab Control 6"(T4."Imaging" ("Tab Control 6")) -> ()
        "wait to reset values" <- w2207
      }
    }
    n994 = local read "Database link"() -> (→"Database link":path)
    n995 = local read "Trap Pos Elements/DMA read"() -> (w1558:u32)
    n996 = local read "Trap AI Elements/DMA read"() -> (w1633:u32)
    n997 = local read "APD Elements/DMA read"() -> (w1599:u32)
    n998 = xnode "Get APD Data"("FPGA VI Reference In"=w1562, "error in"=w1561, "Number of Elements"=w1599, "Timeout (ms)"=-1) -> ("Data"=w1598:u32[], "Elements Remaining"=→"APD FIFO Elements Remaining":u32)  [unwired: 2 out]
    n999 = xnode "Invoke Method"("FPGA VI Reference In"=w1562, "error in"=w1561, "Number of Elements"=w1558, "Timeout (ms)"=-1) -> ("Data"=w1521:u16[], "Elements Remaining"=→"Trap Pos FIFO El Remaining":u32)  [unwired: 2 out]
    n1000 = xnode "Get Trap Data"("FPGA VI Reference In"=w1562, "error in"=w1561, "Number of Elements"=w1633, "Timeout (ms)"=-1 ("Timeout")) -> ("FPGA VI Reference Out"=w1456:T20, "error out"=w1455:errorcluster, "Data"=w1522:i16[], "Elements Remaining"=w1763:u32)
    "FIFO El. Rem." <- w1763
    n1001 = local read "Trap AI FIFO Depth"() -> (w1765:u32)
    n1002 = Subtract(x=w1765, y=w1633) -> (x-y=w1764:u32)
    n1003 = Decimate 1D Array(w1521) -> (w1518:u16[], w1520:u16[], w1519:u16[])
    n1004 = Divide(x=w1763, y=w1764) -> (x/y=w1762:dbl)
    "Buffer Status" <- w1762
    n1005 = To Unsigned Long Integer(number=w1518) -> (unsigned 32bit integer=w1517:u32[])
    n1006 = Join Numbers(hi=w1520, lo=w1519) -> ((hi.lo)=w1516:u32[])
    n1007 = Equal?(x=w1762, y=1.0) -> (x = y?=w1760:bool)
    n1008 = Join Numbers(hi=w1517, lo=w1516) -> ((hi.lo)=w1510:u64[])
    n1009 = call "IR AOM word to freq - vec.vi"("Frequency Word In (double vec)"=w1510) -> ("Frequency Out"=w1557:dbl[])
    n1010 = case "Alert buffer overflow" shown="True" w1760 {
      frame False {
      }
      frame True {
        n1011 = call <vilib>:"Beep.vi"() -> ()  [unwired: 3 in, 9 out]
        "Overflow (data lost)" <- TRUE ("Overflow (data lost)")
      }
    }
    n1012 = Decimate 1D Array(w1557) -> (w1556:dbl[], w1555:dbl[])
    n1013 = Build Array(w1556, w1555) -> (w1554:dbl[][])
    n1014 = local read "Trap Sets"() -> (w1632:u32)
    n1015 = case "Deinterlace trap data, average down PSD" shown="2" w1632 {
      tunnel: w1522 -> [w2294 w2359]
      tunnel: [w2291 w2356] -> w1625
      tunnel: [w2294 w2358] -> w1513
      tunnel: "Detector Type" -> [w2293 w2354]
      tunnel: [w2292 w2357] -> w1624
      tunnel: [w2290 w2355] -> w1738
      frame 1, Default {
        n1016 = Divide(x=w2294, y=3276.7) -> (x/y=w2295:dbl[])
        n1017 = Decimate 1D Array(w2295) -> (w2304:dbl[], w2303:dbl[], w2302:dbl[], w2301:dbl[], w2300:dbl[], w2299:dbl[], w2298:dbl[], w2297:dbl[])
        n1018 = case shown="\"IR-QPD + PSD + FB-QPD position\"" w2293 {
          tunnel: w2304 -> [w2328 w2353]
          tunnel: w2303 -> [w2327 w2352]
          tunnel: w2302 -> [w2312 w2330]
          tunnel: w2301 -> [w2313 w2340]
          tunnel: w2300 -> [w2326 w2351]
          tunnel: w2299 -> [w2325 w2350]
          tunnel: w2298 -> [w2309 w2331]
          tunnel: w2297 -> [w2308 w2329]
          tunnel: [w2307 w2337] -> w2292
          tunnel: [w2306 w2336] -> w2291
          tunnel: [w2305 w2335] -> w2290
          frame "IR-QPD + PSD + FB-QPD", Default {
            w2305 = 0  # Channel pattern
            n1019 = Divide(x=w2328, y=w2313) -> (x/y=w2315:dbl[])
            n1020 = Divide(x=w2327, y=w2313) -> (x/y=w2314:dbl[])
            n1021 = Divide(x=w2326, y=w2309) -> (x/y=w2311:dbl[])
            n1022 = Divide(x=w2325, y=w2308) -> (x/y=w2310:dbl[])
            n1023 = Build Array(w2315, w2314, w2313, w2312, w2311, w2310, w2309, w2308) -> (w2306:dbl[][])
            n1024 = Bundle("T1 Y", "T1 X", "T1 Sum", "FB Sum", "PSD Y", "PSD X", "PSD Y Sum", "PSD X Sum") -> (w2324:T39)  [unwired: 1 out]
            n1025 = Cluster To Array(cluster=w2324) -> (array=w2307:string[])
          }
          frame "IR-QPD + PSD + FB-QPD position" {
            w2335 = 3  # Channel pattern
            n1026 = Negate(x=w2331) -> (-x=w2332:dbl[])
            n1027 = Divide(x=w2353, y=w2340) -> (x/y=w2342:dbl[])
            n1028 = Divide(x=w2352, y=w2340) -> (x/y=w2341:dbl[])
            n1029 = Divide(x=w2351, y=w2331) -> (x/y=w2339:dbl[])
            n1030 = Divide(x=w2350, y=w2332) -> (x/y=w2338:dbl[])
            n1031 = Build Array(w2342, w2341, w2340, w2329, w2330, w2339, w2338, w2331) -> (w2336:dbl[][])
            n1032 = Bundle("T1 Y", "T1 X", "T1 Sum", "FB X", "FB Sum", "PSD Y", "PSD X", "PSD Y Sum") -> (w2349:T39)  [unwired: 1 out]
            n1033 = Cluster To Array(cluster=w2349) -> (array=w2337:string[])
          }
        }
      }
      frame 2 {
        n1034 = case shown="\"IR-QPD + PSD + FB-QPD X position\"" w2354 {
          tunnel: w2359 -> [w2421 w2488 w2559]
          tunnel: [w2360 w2479 w2490] -> w2358
          tunnel: [w2387 w2470 w2537] -> w2357
          tunnel: [w2386 w2433 w2504] -> w2356
          tunnel: [w2380 w2468 w2535] -> w2355
          frame "IR-QPD + PSD + FB-QPD", Default {
            w2380 = 1  # Channel pattern
            # "time average x2 the 4th signal and the 4 psd signals (detection laser)"
            # "deinterlace 3 signals from qpd"
            n1035 = Decimate 1D Array(w2421) -> (w2420:i16[], w2419:i16[], w2385:i16[], w2418:i16[], w2408:i16[], w2406:i16[], w2405:i16[], w2403:i16[])
            n1036 = Decimate 1D Array(w2385) -> (w2384:i16[], w2383:i16[])
            n1037 = Decimate 1D Array(w2420) -> (w2417:i16[], w2389:i16[])
            n1038 = Decimate 1D Array(w2419) -> (w2416:i16[], w2414:i16[])
            n1039 = Decimate 1D Array(w2418) -> (w2415:i16[], w2413:i16[])
            n1040 = call "downsample 1D array - double.vi"("Ave N"=2.0, "Array In"=w2408) -> ("Array Out"=w2407:dbl[])  [unwired: 1 out]
            n1041 = call "downsample 1D array - double.vi"("Ave N"=2.0, "Array In"=w2406) -> ("Array Out"=w2388:dbl[])  [unwired: 1 out]
            n1042 = call "downsample 1D array - double.vi"("Ave N"=2.0, "Array In"=w2405) -> ("Array Out"=w2404:dbl[])  [unwired: 1 out]
            n1043 = call "downsample 1D array - double.vi"("Ave N"=2.0, "Array In"=w2403) -> ("Array Out"=w2402:dbl[])  [unwired: 1 out]
            n1044 = Interleave 1D Arrays(w2417, w2416, w2415, w2389, w2414, w2413, w2384, w2383, w2407, w2388, w2404, w2402) -> (w2401:dbl[])
            n1045 = Divide(x=w2401, y=3276.7) -> (x/y=w2400:dbl[])
            n1046 = Decimate 1D Array(w2400) -> (w2399:dbl[], w2398:dbl[], w2397:dbl[], w2396:dbl[], w2395:dbl[], w2394:dbl[], w2382:dbl[], w2381:dbl[], w2393:dbl[], w2392:dbl[], w2391:dbl[], w2390:dbl[])
            n1047 = Divide(x=w2399, y=w2397) -> (x/y=w2367:dbl[])
            n1048 = Divide(x=w2398, y=w2397) -> (x/y=w2366:dbl[])
            n1049 = Divide(x=w2396, y=w2394) -> (x/y=w2365:dbl[])
            n1050 = Divide(x=w2395, y=w2394) -> (x/y=w2364:dbl[])
            n1051 = Divide(x=w2393, y=w2391) -> (x/y=w2363:dbl[])
            n1052 = Divide(x=w2392, y=w2390) -> (x/y=w2362:dbl[])
            n1053 = Build Array(w2367, w2366, w2397, w2365, w2364, w2394, w2382, w2381, w2363, w2362, w2391, w2390) -> (w2386:dbl[][])
            n1054 = Bundle("T1 Y", "T1 X", "T1 Sum", "T2 Y", "T2 X", "T2 Sum", "T1 FB Sum", "T2 FB Sum", "PSD Y", "PSD X", "PSD Y Sum", "PSD X Sum") -> (w2368:T40)  [unwired: 1 out]
            n1055 = To Word Integer(number=w2401) -> (16bit integer=w2360:i16[])
            n1056 = Cluster To Array(cluster=w2368) -> (array=w2387:string[])
          }
          frame "IR-QPD + PSD + FB-QPD X position" {
            w2468 = 2  # Channel pattern
            # "time average x2 the 3 psd signals (detection laser)"
            # "deinterlace 3 signals from qpds"
            n1057 = Decimate 1D Array(w2488) -> (w2487:i16[], w2486:i16[], w2469:i16[], w2485:i16[], w2431:i16[], w2428:i16[], w2425:i16[], w2456:i16[])
            n1058 = Decimate 1D Array(w2469) -> (w2454:i16[], w2452:i16[])
            n1059 = Decimate 1D Array(w2487) -> (w2484:i16[], w2471:i16[])
            n1060 = Decimate 1D Array(w2486) -> (w2483:i16[], w2481:i16[])
            n1061 = Decimate 1D Array(w2485) -> (w2482:i16[], w2480:i16[])
            n1062 = Decimate 1D Array(w2456) -> (w2455:i16[], w2453:i16[])
            n1063 = call "downsample 1D array - I16.vi"("Ave N"=2.0, "Array In"=w2431) -> ("Array Out"=w2429:i16[])  [unwired: 1 in]
            n1064 = call "downsample 1D array - I16.vi"("Ave N"=2.0, "Array In"=w2425) -> ("Array Out"=w2423:i16[])  [unwired: 1 in]
            n1065 = call "downsample 1D array - I16.vi"("Ave N"=2.0, "Array In"=w2428) -> ("Array Out"=w2426:i16[])  [unwired: 1 in]
            n1066 = Interleave 1D Arrays(w2484, w2483, w2482, w2471, w2481, w2480, w2455, w2454, w2453, w2452, w2429, w2426, w2423) -> (w2479:i16[])
            n1067 = Divide(x=w2479, y=3276.7) -> (x/y=w2478:dbl[])
            n1068 = Decimate 1D Array(w2478) -> (w2477:dbl[], w2476:dbl[], w2475:dbl[], w2474:dbl[], w2473:dbl[], w2472:dbl[], w2444:dbl[], w2442:dbl[], w2441:dbl[], w2439:dbl[], w2438:dbl[], w2437:dbl[], w2434:dbl[])
            n1069 = Negate(x=w2434) -> (-x=w2432:dbl[])
            n1070 = Divide(x=w2438, y=w2434) -> (x/y=w2436:dbl[])
            n1071 = Divide(x=w2437, y=w2432) -> (x/y=w2435:dbl[])
            n1072 = Divide(x=w2477, y=w2475) -> (x/y=w2460:dbl[])
            n1073 = Divide(x=w2476, y=w2475) -> (x/y=w2459:dbl[])
            n1074 = Divide(x=w2474, y=w2472) -> (x/y=w2458:dbl[])
            n1075 = Divide(x=w2473, y=w2472) -> (x/y=w2457:dbl[])
            n1076 = Divide(x=w2444, y=w2442) -> (x/y=w2443:dbl[])
            n1077 = Divide(x=w2441, y=w2439) -> (x/y=w2440:dbl[])
            n1078 = Build Array(w2460, w2459, w2475, w2458, w2457, w2472, w2443, w2442, w2440, w2439, w2436, w2435, w2434) -> (w2433:dbl[][])
            n1079 = Bundle("T1 Y", "T1 X", "T1 Sum", "T2 Y", "T2 X", "T2 Sum", "T1 FB X", "T1 FB Sum", "T2 FB X", "T2 FB Sum", "PSD Y", "PSD X", "PSD Y Sum") -> (w2461:T41)  [unwired: 1 out]
            n1080 = Cluster To Array(cluster=w2461) -> (array=w2470:string[])
          }
          frame "IR-QPD + PSD + FB-QPD XY positions" {
            w2535 = 4  # Channel pattern
            # "time average x2 the 3 psd signals (detection laser)"
            # "deinterlace 3 signals from qpds"
            n1081 = Decimate 1D Array(w2559) -> (w2558:i16[], w2557:i16[], w2536:i16[], w2556:i16[], w2502:i16[], w2548:i16[], w2547:i16[], w2524:i16[])
            n1082 = Decimate 1D Array "Feedback Sum"(w2536) -> (w2520:i16[], w2518:i16[])
            n1083 = Decimate 1D Array "QPD Y"(w2558) -> (w2555:i16[], w2538:i16[])
            n1084 = Decimate 1D Array "QPD X"(w2557) -> (w2554:i16[], w2552:i16[])
            n1085 = Decimate 1D Array "Feedback Y"(w2502) -> (w2501:i16[], w2500:i16[])
            n1086 = Decimate 1D Array "QPD Sum"(w2556) -> (w2553:i16[], w2551:i16[])
            n1087 = Decimate 1D Array "Feedback X"(w2524) -> (w2521:i16[], w2519:i16[])
            n1088 = call "downsample 1D array - double.vi"("Ave N"=2.0, "Array In"=w2548) -> ("Array Out"=w2523:dbl[])  [unwired: 1 out]
            n1089 = call "downsample 1D array - double.vi"("Ave N"=2.0, "Array In"=w2547) -> ("Array Out"=w2522:dbl[])  [unwired: 1 out]
